vi "update_website_text.vi"(4 "Refresh Time [seconds]":dbl=1.0 min=0.0 step=0.1 format="%#.1g", 6 "Font Size":u16=200, 7 "Text":string, 8 "error in":errorcluster, 9 "Endpoint":string, 10 "Port":u16=1683, 11 "Hostname or IP Address":string="127.0.0.1") -> (0 "error out":errorcluster)   [LabVIEW 2010]
uses:
  <vilib>/httpClient/LabVIEWHTTPClient.lvlib
  <vilib>/httpClient/PUTBuffer.vi
  <vilib>/regexp/Match Regular Expression.xnode
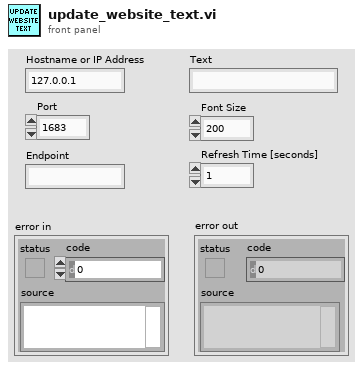
[diagram p1: front panel]
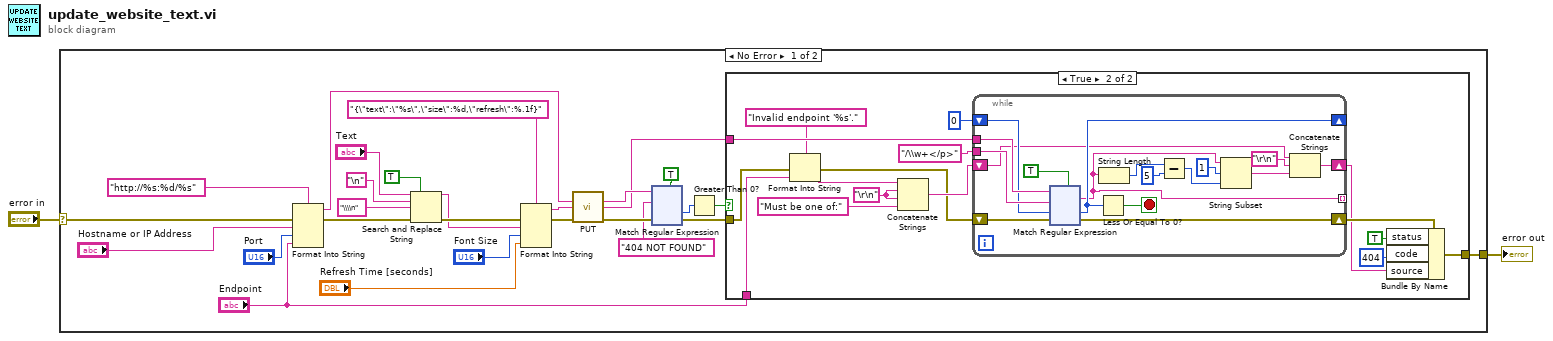
[diagram p0: block diagram]
diagram:
  n1 = case shown="No Error" "error in" {
    selector: "error in" -> [w13 w292]
    tunnel: [w5 w292] -> w2
    frame No Error {
      n2 = Format Into String(format string="http://%s:%d/%s", error in=w13, "Hostname or IP Address", "Port", "Endpoint") -> (resulting string=w26:string, error out=w14:errorcluster)  [unwired: 1 in]
      n3 = Search and Replace String(replace all?=TRUE ("replace all? (F)"), input string="Text", search string="\n", replace string="\\\\n" ("string"), error in=w14) -> (result string=w15:string, error out=w20:errorcluster)  [unwired: 3 in, 2 out]
      n4 = Format Into String(format string="{\"text\":\"%s\",\"size\":%d,\"refresh\":%.1f}", error in=w20, w15, "Font Size", "Refresh Time [seconds]") -> (resulting string=w23:string, error out=w19:errorcluster)  [unwired: 1 in]
      n5 = call-poly <vilib>:"PUT.vi"("url"=w26, "buffer"=w23, "error in (no error)"=w19) -> ("headers"=w7:string, "body"=w4:string, "error out"=w11:errorcluster)  [unwired: 9 in, 1 out]
      n6 = xnode "Match Regular Expression"("input string"=w7, "regular expression"="404 NOT FOUND", "error in"=w11, "multiline? (F)"=TRUE) -> ("offset past match"=w9:i32, "error out"=w6:errorcluster)  [unwired: 2 in, 3 out]
      n7 = Greater Than 0?(x=w9) -> (x > 0?=w8:bool)
      n8 = case shown="True" w8 {
        tunnel: w6 -> [w144 w152]
        tunnel: [w144 w148] -> w5
        tunnel: w4 -> [_ w160]
        tunnel: "Endpoint" -> [_ w153]
        frame False {
        }
        frame True {
          w155 = "\r\n"
          n9 = Format Into String(format string="Invalid endpoint '%s'.", error in=w152, w153) -> (resulting string=w150:string, error out=w151:errorcluster)  [unwired: 1 in]
          n10 = Concatenate Strings(w150, w155, w155, "Must be one of:") -> (w156:string)
          n11 = while {
            tunnel: "/\\w+</p>" ("regular expression") -> [w175]
            tunnel: w160 -> [w177]
            shift-right: [w172] -> _
            shift-left: 0 -> [w174]
            shift-right: [w170] -> w147
            shift-left: w156 -> [w171]
            shift-right: [w162] -> w149
            shift-left: w151 -> [w163]
            tunnel: [w161] -> _ mode=indexing
            stop <- w173 stop-if-true
            n12 = xnode "Match Regular Expression"("input string"=w177, "regular expression"=w175, "offset (0)"=w174, "error in"=w163, "multiline? (F)"=TRUE) -> ("whole match"=w161:string, "offset past match"=w172:i32, "error out"=w162:errorcluster)  [unwired: 1 in, 2 out]
            n13 = Less Or Equal To 0?(x=w172) -> (x <= 0?=w173:bool)
            n14 = String Length(string=w161) -> (length=w167:i32)
            n15 = Subtract(x=w167, y=5) -> (x-y=w165:i32)
            n16 = String Subset(string=w161, offset (0)=1, length (rest)=w165) -> (substring=w164:string)
            n17 = Concatenate Strings(w171, "\r\n", w164) -> (w170:string)
          }
          n18 = Bundle By Name(cluster=w149, "status"=TRUE, "code"=404, "source"=w147) -> (w148:errorcluster)
        }
      }
    }
    frame Error {
    }
  }
  "error out" <- w2
